vi "Get Shared Assets Paths.vi"() -> (1 "RTs Only":T1, 2 "BC Only":T1, 3 "BC and RTs":T1)   [LabVIEW 2020]
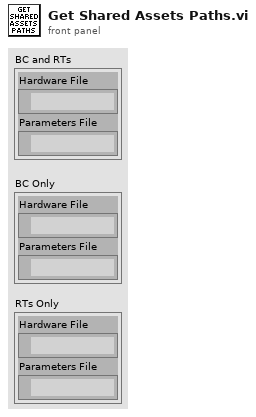
[diagram p1: front panel]
types:
  T1 = cluster{"Hardware File":path, "Parameters File":path}
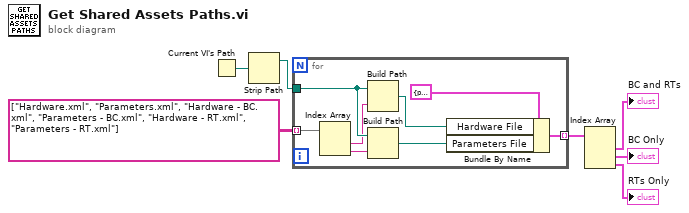
[diagram p0: block diagram]
diagram:
  n1 = Current VI's Path() -> (path=w7:path)
  n2 = Strip Path(path=w7) -> (stripped path=w6:path)  [unwired: 1 out]
  n3 = for {
    tunnel: w6 -> [w14]
    tunnel: string[][] [["Hardware.xml", "Parameters.xml"], ["Hardware - BC.xml", "Parameters - BC.xml"], ["Hardware - RT.xml", "Parameters - RT.xml"]] -> [w15] mode=indexing
    tunnel: [w8] -> w4 mode=indexing
    n4 = Index Array(array=w15) -> (element #1=w12:string, element #2=w13:string)  [unwired: 2 in]
    n5 = Build Path(base path=w14, name or relative path=w12) -> (appended path=w10:path)
    n6 = Build Path(base path=w14, name or relative path=w13) -> (appended path=w9:path)
    n7 = Bundle By Name(cluster=T1 {"Hardware File"=path "", "Parameters File"=path ""}, "Hardware File"=w10, "Parameters File"=w9) -> (w8:T1)
  }
  n8 = Index Array(array=w4) -> (element #1=→"BC and RTs":T1, element #2=→"BC Only":T1, element #3=→"RTs Only":T1)  [unwired: 3 in]
